vi "Read Working Path.vi"() -> (3 "Working Path":path)   [LabVIEW 2020, in "SimpleDependencyInspector.lvlib"]
uses:
  SimpleDependencyInspector.lvlib
  <resource>/dialog/lvconfig.llb/LV Config Read Pathlist.vi
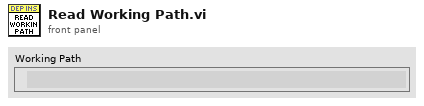
[diagram p1: front panel]
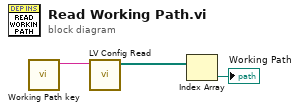
[diagram p0: block diagram]
diagram:
  n1 = call "Working Path key.vi"() -> ("String"=w1:string)  [unwired: 11 in]
  n2 = call-poly <resource>:"LV Config Read.vi"("key"=w1) -> ("value"=w2:path[])  [unwired: 4 in, 2 out]
  n3 = Index Array(array=w2) -> (element=→"Working Path":path)  [unwired: 1 in]
